vi "rad_Retrieve Image Wrapper.vi"(5 "Password":string, 7 "Deployment Notifiers":T6, 8 "error in (no error)":errorcluster, 9 "AppImage Properties":T3, 10 "image file path":path, 11 "Target settings":T1={"Hostname"="", "Serial number"="", "Product name"="", "Product code"=0, "System status"="", "Credential type"=enum."None/Unlocked", "User added?"=FALSE, "Primary NIC"={"MAC address"="", "IP Address Request Mode"=2, "IP address"="", "Subnet mask"="", "Gateway"="", "DNS server"=""}} {"Primary NIC"."IP Address Request Mode" items=["Static"=1, "DHCP/Link-Local"=2, "Link-Local Only"=4, "DHCP Only"=8]}) -> (0 "error out":errorcluster, 3 "Canceled":bool)   [LabVIEW 2020]
uses:
  <vilib>/nisyscfg/nisyscfg.lvlib
  <vilib>/nisyscfg/Software 1.2.ctl
  <vilib>/nisyscfg/Component Type.ctl
  <vilib>/nisyscfg/Create System Image (Folder).vi
  <vilib>/nisyscfg/Close (System).vi
  TypeDefs/rad_Deployment Status Data Type.ctl
  TypeDefs/rad_Deployment Progress Data Type.ctl
  TypeDefs/rad_Deployment Notifiers.ctl
  TypeDefs/rad_FPGA Flash Properties.ctl
  TypeDefs/rad_FPGA Properties.ctl
  TypeDefs/rad_Application Image Properties.ctl
  Targets/TypeDefs/rad_Target Information.ctl
  Targets/TypeDefs/rad_Target Network Settings.ctl
panel:
  in  "Stop Checking for Events":bool
  out "Progress":T7 scale=0.0..100.0
  out "Status":string
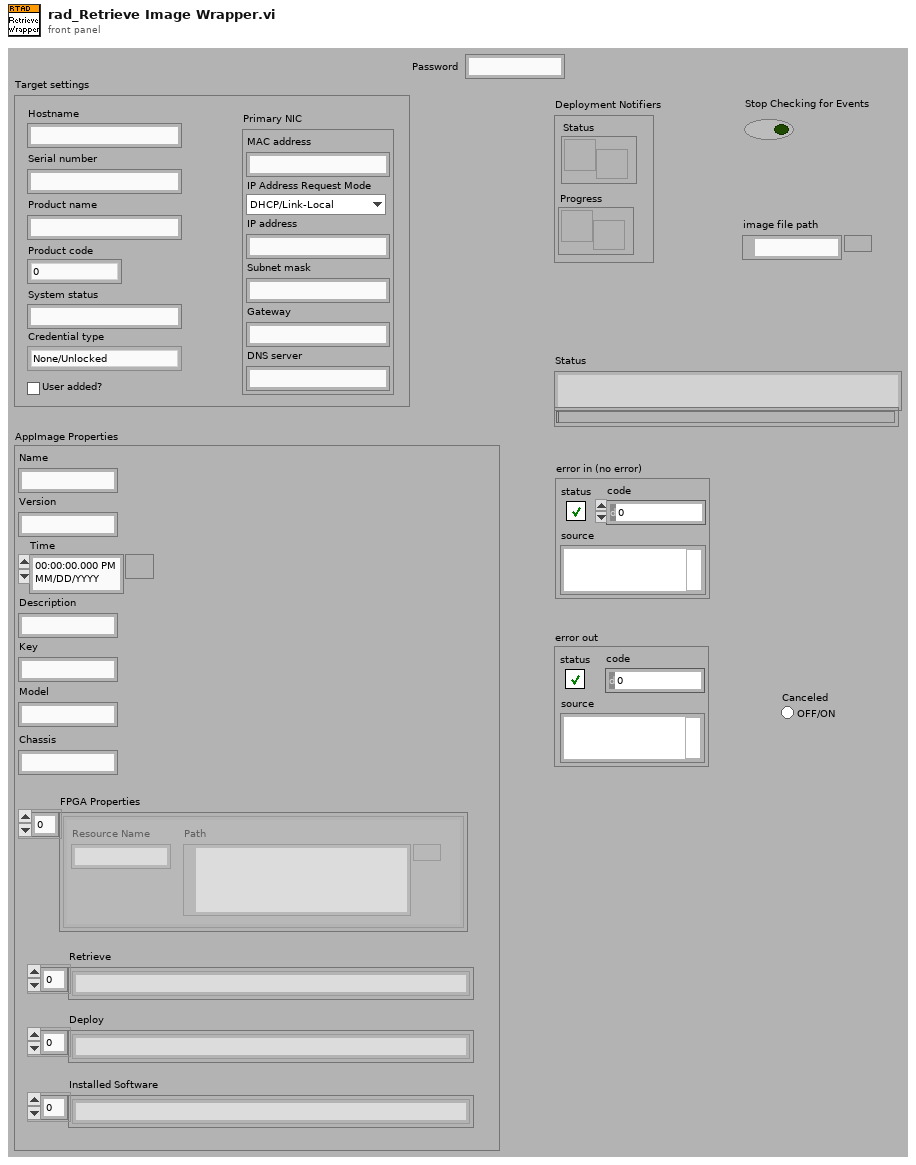
[diagram p1: front panel]
types:
  T1 = typedef "rad_Target Information.ctl" = cluster{"Hostname":string, "Serial number":string, "Product name":string, "Product code":i32, "System status":string, "Credential type":enum16{"None/Unlocked", "FTP Password", "NIAuth Credentials"}, "User added?":bool, "Primary NIC":T2}
  T2 = typedef "rad_Target Network Settings.ctl" = cluster{"MAC address":string, "IP Address Request Mode":i32, "IP address":string, "Subnet mask":string, "Gateway":string, "DNS server":string}
  T3 = typedef "rad_Application Image Properties.ctl" = cluster{"Name":string, "Version":string, "Time":timestamp, "Description":string, "Key":string, "Chassis":string, "FPGA Properties":T4, "Model":string, "Retrieve":string[], "Deploy":string[], "Installed Software":string[]}
  T4 = typedef "rad_FPGA Properties.ctl" = T5[]
  T5 = typedef "rad_FPGA Flash Properties.ctl" = cluster{"Resource Name":string, "Path":path}
  T6 = typedef "rad_Deployment Notifiers.ctl" = cluster{"Status":refnum<notifier>, "Progress":refnum<notifier>}
  T7 = typedef "rad_Deployment Progress Data Type.ctl" = i8
  T8 = typedef "nisyscfg.lvlib/Software 1.2.ctl" = cluster{"title":string, "description":string, "ID":string, "version":string, "component type":T9}
  T9 = typedef "nisyscfg.lvlib/Component Type.ctl" = u32
  T10 = enum32{"state changed", "beginning restart", "getting file", "putting file", "creating directory", "deleting file", "deleting directory", "enumerating file system", "renaming file", "current component", "operation progress", "downloading file", "unpacking file", "running install script", "creating image", "validating image", "applying image", "beginning format", "completing format"}
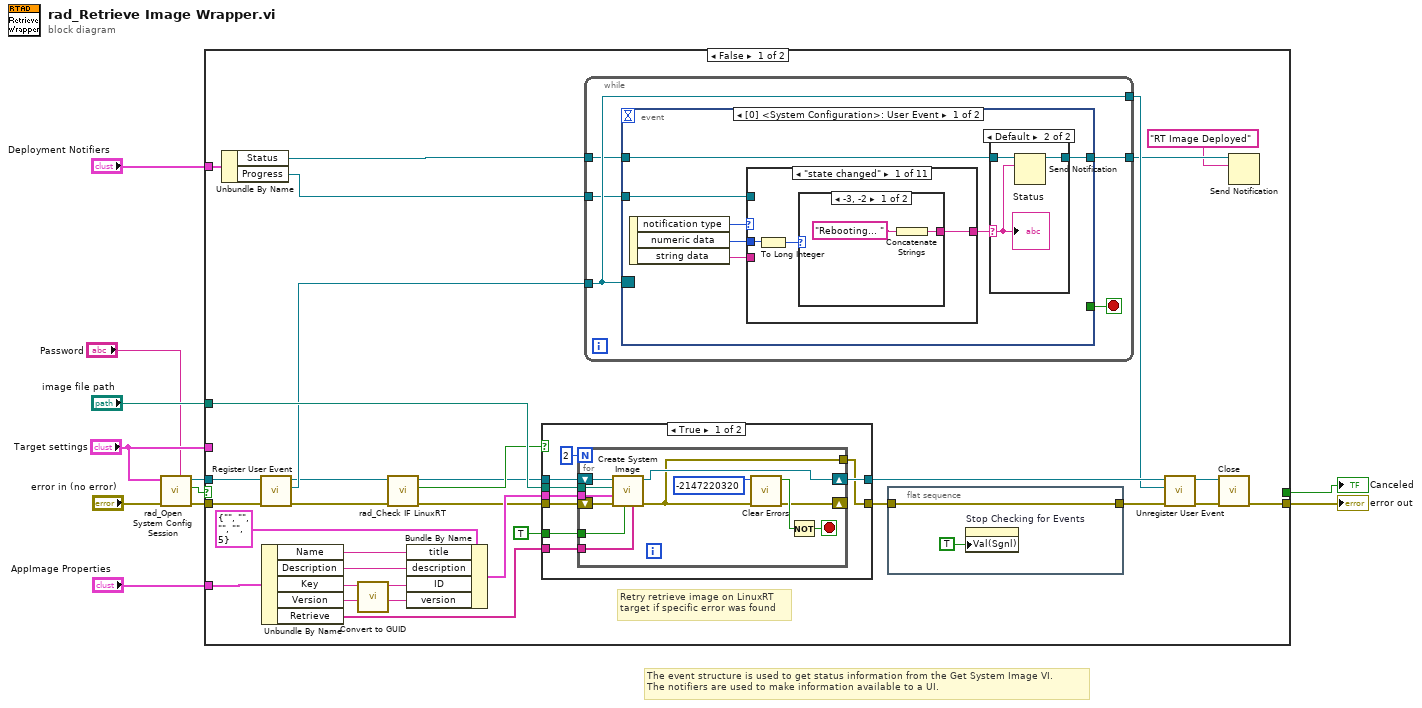
[diagram p0: block diagram]
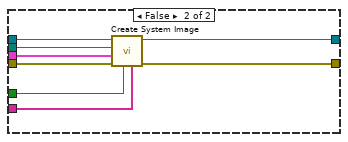
[diagram p2: hidden frame]
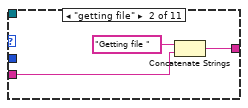
[diagram p5: hidden frame]
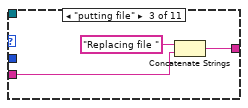
[diagram p6: hidden frame]
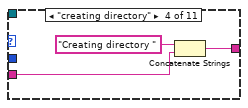
[diagram p7: hidden frame]
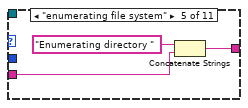
[diagram p8: hidden frame]
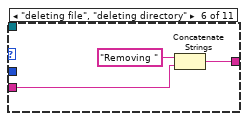
[diagram p9: hidden frame]
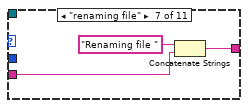
[diagram p10: hidden frame]
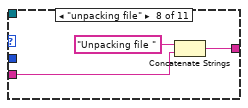
[diagram p11: hidden frame]
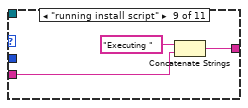
[diagram p12: hidden frame]
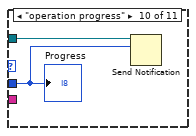
[diagram p13: hidden frame]
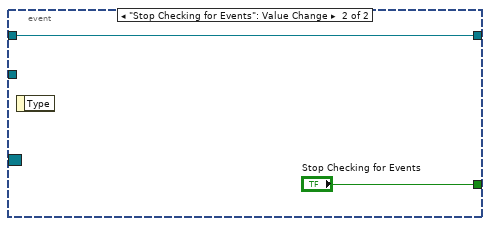
[diagram p15: hidden frame]
diagram:
  # "The event structure is used to get status information from the Get System Image VI. \nThe notifiers are used to make information available to a UI."
  n1 = call "rad_Open System Config Session.vi"("Password"="Password", "error in (no error)"="error in (no error)", "Target settings"="Target settings") -> ("error out"=w4:errorcluster, "Cancelled"=w3:bool, "Session out"=w5:refnum<k21>)  [unwired: 5 in, 1 out]
  n2 = case shown="False" w3 {
    selector: w3 -> [_ w123]
    tunnel: [w42 w124] -> w9
    tunnel: "image file path" -> [w41 _]
    tunnel: w5 -> [w40 _]
    tunnel: w4 -> [w39 w124]
    tunnel: "Deployment Notifiers" -> [w26 _]
    tunnel: "AppImage Properties" -> [w25 _]
    tunnel: [_ w123] -> w7
    tunnel: "Target settings" -> [_ _]
    frame False {
      # "Retry retrieve image on LinuxRT\ntarget if specific error was found"
      n3 = Unbundle By Name(w26) -> ("Status"=w28:refnum<notifier>, "Progress"=w27:refnum<notifier>)
      n4 = call <vilib>:"Register User Event.vi"("error in (no error)"=w39, "Session in"=w40) -> ("error out"=w15:errorcluster, "Event Registration out"=w38:refnum<event-registration>, "Session out"=w16:refnum<k21>)  [unwired: 7 in]
      n5 = Unbundle By Name(w25) -> ("Name"=w23:string, "Description"=w22:string, "Key"=w19:string, "Version"=w21:string, "Retrieve"=w17:string[])
      n6 = call "Convert to GUID.vi"("Key"=w19) -> ("GUID"=w18:string)  [unwired: 10 in]
      n7 = call "rad_Check IF LinuxRT.vi"("Error In"=w15, "System Session In"=w16) -> ("Error Out"=w12:errorcluster, "Target is LinuxRT?"=w14:bool, "System Session Out"=w13:refnum<k21>)  [unwired: 5 in, 2 out]
      n8 = Bundle By Name(cluster=T8 {"title"="", "description"="", "ID"="", "version"="", "component type"=5} ("image metadata"), "title"=w23, "description"=w22, "ID"=w18, "version"=w21) -> (w20:T8)
      n9 = case shown="True" w14 {
        tunnel: w41 -> [w51 w71]
        tunnel: w13 -> [w50 w70]
        tunnel: w12 -> [w49 w69]
        tunnel: [w48 w68] -> w35
        tunnel: [w43 w67] -> w33
        tunnel: TRUE ("overwrite (F)") -> [w47 w66]
        tunnel: w20 -> [w46 w65]
        tunnel: w17 -> [w45 w64]
        frame True {
          n10 = for {
            N: 2 -> [_]
            tunnel: w51 -> [w63]
            tunnel: w47 -> [w60]
            tunnel: w46 -> [w59]
            shift-right: [w55] -> w48
            shift-left: w50 -> [w62]
            shift-right: [w53] -> _
            shift-left: w49 -> [w61]
            tunnel: w45 -> [w58]
            tunnel: [w54] -> w43
            stop <- w57 stop-if-true
            n11 = call-poly <vilib>:"Create System Image.vi"("File and Directory Blacklist"=w58, "Overwrite (F)"=w60, "error in (no error)"=w61, "Image Metadata in"=w59, "Destination Folder"=w63, "Session in"=w62) -> ("error out"=w54:errorcluster, "Session out"=w55:refnum<k21>)  [unwired: 3 in, 1 out]
            n12 = call <vilib>:"Clear Errors.vi"("error in (no error)"=w54, "specific error code to clear (0: all)"=-2147220320) -> ("error out"=w53:errorcluster, "specific error cleared?"=w56:bool)  [unwired: 4 in]
            n13 = Not(x=w56) -> (.not. x?=w57:bool)
          }
        }
        frame False {
          n14 = call-poly <vilib>:"Create System Image.vi"("File and Directory Blacklist"=w64, "Overwrite (F)"=w66, "error in (no error)"=w69, "Image Metadata in"=w65, "Destination Folder"=w71, "Session in"=w70) -> ("error out"=w67:errorcluster, "Session out"=w68:refnum<k21>)  [unwired: 3 in, 1 out]
        }
      }
      n15 = while {
        tunnel: w38 -> [w78]
        tunnel: [w78] -> w34
        tunnel: w28 -> [w76]
        tunnel: [w75] -> w31
        tunnel: w27 -> [w74]
        stop <- w77 stop-if-true
        n16 = event shown="[0] <System Configuration>: User Event" {
          selector: w78 -> [_ _]
          dyn-events: _ -> [_ _]
          timeout: _ -> [_ _]
          tunnel: [_ "Stop Checking for Events"] -> w77
          tunnel: w76 -> [w81 w121]
          tunnel: [w80 w121] -> w75
          tunnel: w74 -> [w79 _]
          event User Event {
            n17 = event-data() -> ("notification type"=w85:T10, "numeric data"=w83:u32, "string data"=w84:string)  [unwired: 1 in]
            n18 = case shown="\"state changed\"" w85 {
              tunnel: [w90 w95 w98 w101 w104 w107 w110 w113 w116 _ _] -> w82
              tunnel: w84 -> [_ w96 w99 w102 w105 w108 w111 w114 w117 _ _]
              tunnel: w83 -> [w92 _ _ _ _ _ _ _ _ w119 _]
              tunnel: w79 -> [_ _ _ _ _ _ _ _ _ w120 _]
              frame "state changed" {
                n19 = To Long Integer(number=w92) -> (32bit integer=w91:i32)
                n20 = case shown="-3, -2" w91 {
                  tunnel: [w93 _] -> w90
                  frame -3, -2 {
                    n21 = Concatenate Strings("Rebooting... ") -> (w93:string)
                  }
                  frame Default {
                  }
                }
              }
              frame "getting file" {
                n22 = Concatenate Strings("Getting file " ("Status"), w96) -> (w95:string)
              }
              frame "putting file" {
                n23 = Concatenate Strings("Replacing file " ("Status"), w99) -> (w98:string)
              }
              frame "creating directory" {
                n24 = Concatenate Strings("Creating directory " ("Status"), w102) -> (w101:string)
              }
              frame "enumerating file system" {
                n25 = Concatenate Strings("Enumerating directory " ("Status"), w105) -> (w104:string)
              }
              frame "deleting file", "deleting directory" {
                n26 = Concatenate Strings("Removing " ("Status"), w108) -> (w107:string)
              }
              frame "renaming file" {
                n27 = Concatenate Strings("Renaming file " ("Status"), w111) -> (w110:string)
              }
              frame "unpacking file" {
                n28 = Concatenate Strings("Unpacking file " ("Status"), w114) -> (w113:string)
              }
              frame "running install script" {
                n29 = Concatenate Strings("Executing " ("Status"), w117) -> (w116:string)
              }
              frame "operation progress" {
                n30 = Send Notification(notification=w119, notifier=w120) -> ()  [unwired: 1 in, 2 out]
                "Progress" <- w119
              }
              frame Default {
              }
            }
            n31 = case shown="Default" w82 {
              selector: w82 -> [_ w88]
              tunnel: w81 -> [w86 w89]
              tunnel: [w86 w87] -> w80
              frame "" {
              }
              frame Default {
                n32 = Send Notification(notification=w88, notifier=w89) -> (notifier out=w87:refnum<notifier>)  [unwired: 1 in, 1 out]
                "Status" <- w88
              }
            }
          }
          event "Stop Checking for Events": Value Change {
            n33 = event-data() -> ()  [unwired: 1 in, 1 out]
          }
        }
      }
      n34 = flat-sequence {
        tunnel: w33 -> [w73]
        tunnel: [w73] -> w32
        frame #0 {
          n35 = property on="Stop Checking for Events" class="Bool (strict)"("Val(Sgnl)"=TRUE ("Stop Checking for Events")) -> ()  [unwired: 2 in, 2 out]
        }
      }
      n36 = call <vilib>:"Unregister User Event.vi"("error in (no error)"=w32, "Event Registration in"=w34, "Session in"=w35) -> ("error out"=w36:errorcluster, "Session out"=w37:refnum<k21>)  [unwired: 7 in]
      n37 = call-poly <vilib>:"Close.vi"("error in (no error)"=w36, "Session in"=w37) -> ("error out"=w42:errorcluster)  [unwired: 9 in]
      n38 = Send Notification(notification="RT Image Deployed", notifier=w31) -> ()  [unwired: 1 in, 2 out]
    }
    frame True {
    }
  }
  "error out" <- w9
  "Canceled" <- w7
